vi "Set Display On Off.vi"(8 "Error In":errorcluster, 10 "Display On/Off":enum8{"Off", "On"}(ring), 11 "LINX Resource 2":T1) -> (0 "Error Out":errorcluster, 3 "LINX Resource":T1)   [LabVIEW 2013, in "LVH-LINX.lvlib" / "SSD1306.lvlib"]
doc: "Turn the SSD1306 display on or off."
uses:
  <vilib>/LabVIEW Hacker/LINX/Public/Sensors/Display/SSD1306/SSD1306.lvlib
  <vilib>/LabVIEW Hacker/LINX/Private/Type Defs/LINX Ref.ctl
  <vilib>/LabVIEW Hacker/LINX/Private/Type Defs/Platform.ctl
  <vilib>/LabVIEW Hacker/LINX/Private/Type Defs/Interface.ctl
  <vilib>/LabVIEW Hacker/LINX/Private/Device/Type Defs/LINX Device Config.ctl
  <vilib>/LabVIEW Hacker/LINX/Private/Device/Type Defs/TCP Config.ctl
  <vilib>/LabVIEW Hacker/LINX/Private/Type Defs/Device Family.ctl
  <vilib>/LabVIEW Hacker/LINX/Public/Sensors/Display/SSD1306/Private/SSD1306 FGV State.ctl
  <vilib>/LabVIEW Hacker/LINX/Public/Peripherals/Digital/Digital Write 1 Chan.vi
  <vilib>/LabVIEW Hacker/LINX/LVH-LINX.lvlib
  <vilib>/LabVIEW Hacker/LINX/Private/Device/Device.lvlib
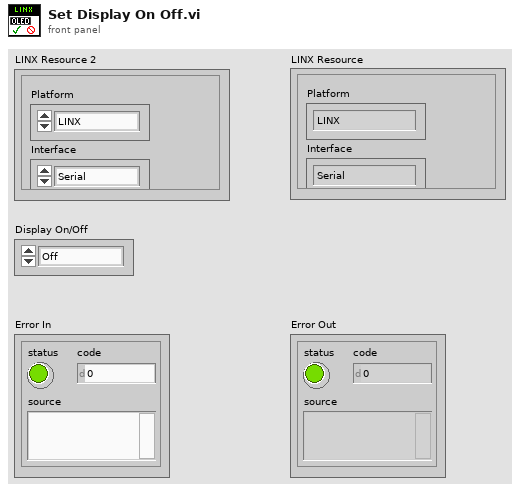
[diagram p1: front panel]
types:
  T1 = typedef "LVH-LINX.lvlib/LINX Ref.ctl" = cluster{"Platform":T2, "Interface":T3, "LINX Device Config":T4}
  T2 = typedef "LVH-LINX.lvlib/Platform.ctl" = enum16{"LINX", "myRIO"}
  T3 = typedef "LVH-LINX.lvlib/Interface.ctl" = enum16{"Serial", "TCP"}
  T4 = typedef "LVH-LINX.lvlib/Device.lvlib/LINX Device Config.ctl" = cluster{"Interface":T3, "COM Port":refnum<visa-resource-name>, "TCP Configuration":T5, "Device Family":T6, "Device ID":u8, "Device Name":string, "TCP Ref":refnum<k5>}
  T5 = typedef "LVH-LINX.lvlib/Device.lvlib/TCP Config.ctl" = cluster{"IP Address":string, "Port":u16}
  T6 = typedef "LVH-LINX.lvlib/Device Family.ctl" = enum8{"National Instruments", "Digilent", "Arduino"}
  T7 = typedef "LVH-LINX.lvlib/SSD1306.lvlib/SSD1306 FGV State.ctl" = enum16{"Init", "Set", "Get"}
  T8 = typedef "LVH-LINX.lvlib/SSD1306.lvlib/SSD1306 Config.ctl" = cluster{"SPI Channel (0)":u8, "VDD Channel":u8, "VBAT Channel":u8, "RESET Channel":u8, "DC Channel":u8, "SPI CS (3)":u8}
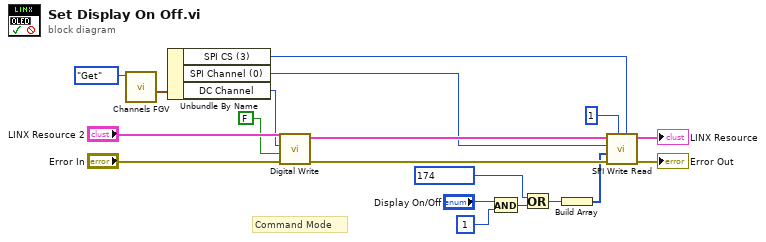
[diagram p0: block diagram]
diagram:
  # "Command Mode"
  n1 = call <vilib>:"Channels FGV.vi"("SSD1306 FGV State"=SSD1306_FGV_State."Get") -> ("SSD1306 Channels"=w16:T8)  [unwired: 10 in]
  n2 = Unbundle By Name(w16) -> ("SPI CS (3)"=w1:u8, "SPI Channel (0)"=w11:u8, "DC Channel"=w15:u8)
  n3 = call-poly <vilib>:"Digital Write.vi"("Error In"="Error In", "Output Value"=FALSE, "DO Channel"=w15, "LINX Resource"="LINX Resource 2") -> ("Error Out"=w12:errorcluster, "LINX Resource"=w13:T1)  [unwired: 6 in]
  n4 = And(x="Display On/Off", y=u8 1 ("SPI Frame Size")) -> (x .and. y?=w4:u8)
  n5 = Or(x=u8 174, y=w4) -> (x .or. y?=w2:u8)
  n6 = Build Array(w2) -> (w7:u8[])
  n7 = call <vilib>:"SPI Write Read.vi"("CS Pin (10)"=w1, "SPI Frame Size"=u8 1, "Error In"=w12, "Data"=w7, "SPI Channel (0)"=w11, "LINX Resource"=w13) -> ("Error Out"=→"Error Out":errorcluster, "LINX Resource"=→"LINX Resource":T1)  [unwired: 3 in, 1 out]
